vi "RectangleToArray.vi"(11 "Optional Rectangle":T1) -> (3 "Array":i32[](array[numeric]))   [LabVIEW 2020, in "OpenLvVision_Image.lvlib" / "DataAccess.lvlib"]
uses:
  DataAccess.lvlib
  TypeDef/RectangleI32.ctl
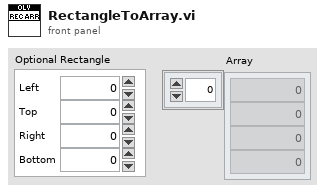
[diagram p1: front panel]
types:
  T1 = typedef "OpenLvVision_Image.lvlib/DataAccess.lvlib/RectangleI32.ctl" = cluster{"Left":i32, "Top":i32, "Right":i32, "Bottom":i32}
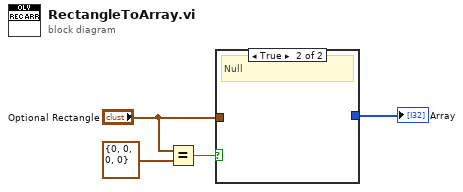
[diagram p0: block diagram]
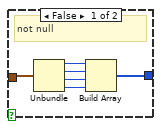
[diagram p2: hidden frame]
diagram:
  n1 = Equal?(x="Optional Rectangle", y=T1 {"Left"=0, "Top"=0, "Right"=0, "Bottom"=0} ("Optional Rectangle")) -> (x = y?=w3:bool)
  n2 = case shown="True" w3 {
    tunnel: "Optional Rectangle" -> [w10 _]
    tunnel: [w5 _] -> w1
    frame False {
      # "not null"
      n3 = Unbundle(w10) -> ("Left"=w9:i32, "Top"=w8:i32, "Right"=w7:i32, "Bottom"=w6:i32)
      n4 = Build Array(w9, w8, w7, w6) -> (w5:i32[])
    }
    frame True {
      # "Null"
    }
  }
  "Array" <- w1
